vi "Y_AxisMotorControlSetupAndHome.vi"(9 "Serial Settings":T1={"baud rate"=57600, "data bits"=8, "parity"=enum."None", "stop bits"=10, "flow control"=0} {"flow control" items=["None"=0, "XON/XOFF"=1, "RTS/CTS"=2, "DTR/DSR"=4]; "stop bits" items=["1.0"=10, "1.5"=15, "2.0"=20]; "data bits" min=5 max=8 step=1; "baud rate" items=["75"=75, "110"=110, "134"=134, "150"=150, "300"=300, "600"=600, "1200"=1200, "1800"=1800, "2400"=2400, "4800"=4800, "7200"=7200, "9600"=9600, "14400"=14400, "19200"=19200, "28800"=28800, "38400"=38400, "56000"=56000, "57600"=57600, "115200"=115200, "128000"=128000, "230400"=230400]}, 11 "VISA Refnum in":refnum<visa-resource-name>="COM3") -> ()   [LabVIEW 2020]
uses:
  C:/Program Files/National Instruments/LabVIEW 2020/examples/Instrument IO/Serial/support/Serial - Settings.ctl
  <vilib>/Instr/_visa.llb/VISA Configure Serial Port (Instr).vi
panel:
  out "Finished":bool
  out "Status Array":bool[](array[boolean])
  out "Limit Switch Status":i32 format="%b"
  out "Buffer":string
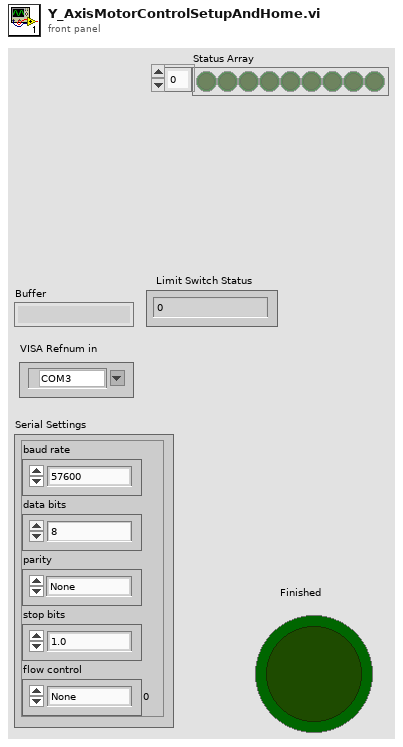
[diagram p1: front panel]
types:
  T1 = typedef "Serial - Settings.ctl" = cluster{"baud rate":u32, "data bits":u16, "parity":enum16{"None", "Odd", "Even", "Mark", "Space"}, "stop bits":u16, "flow control":u16}
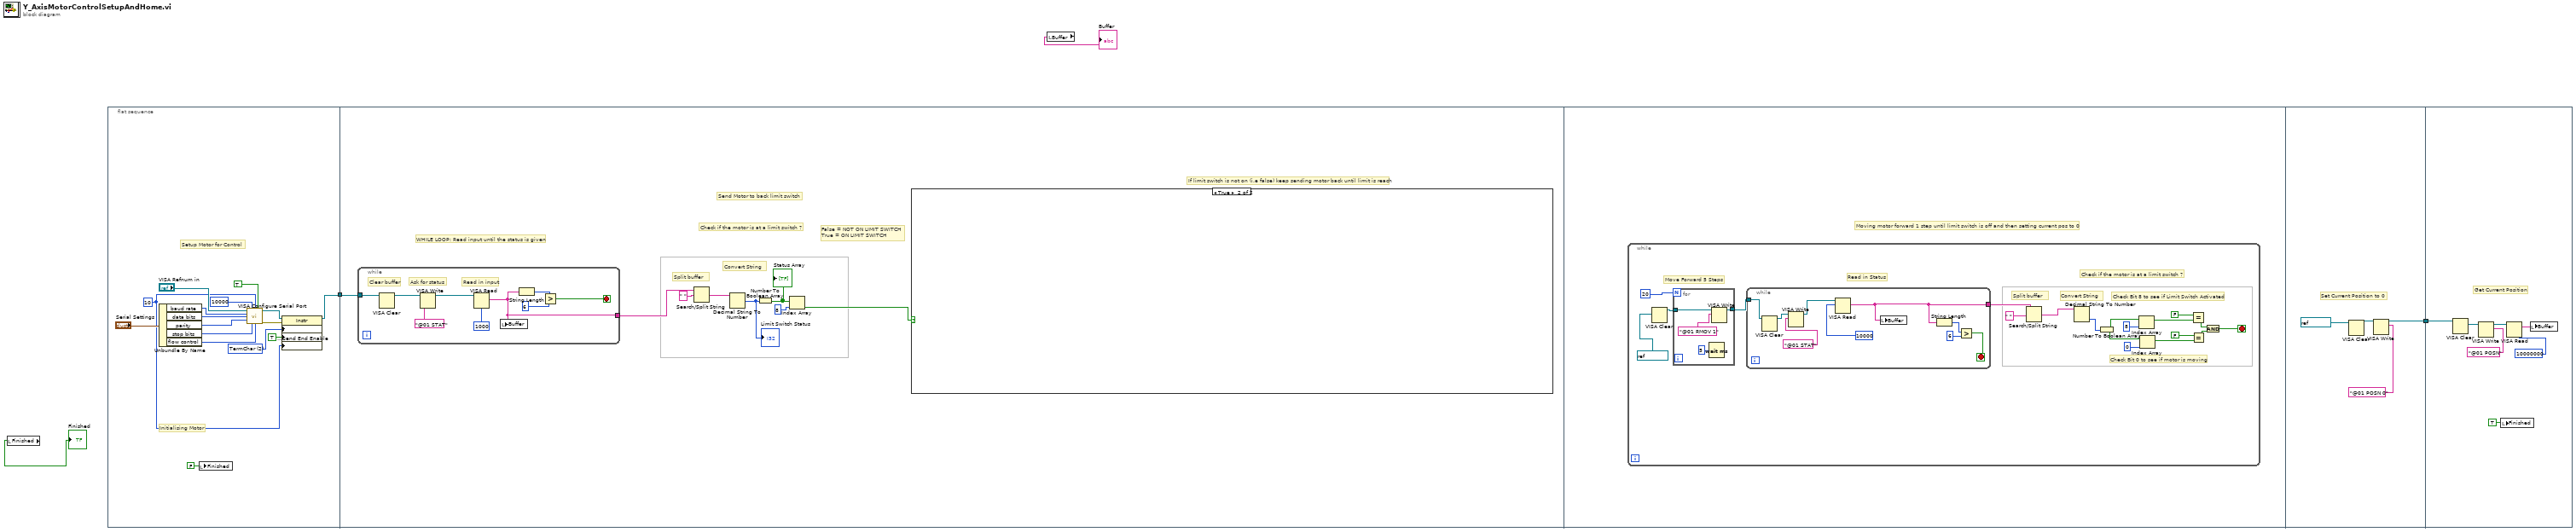
[diagram p0: block diagram]
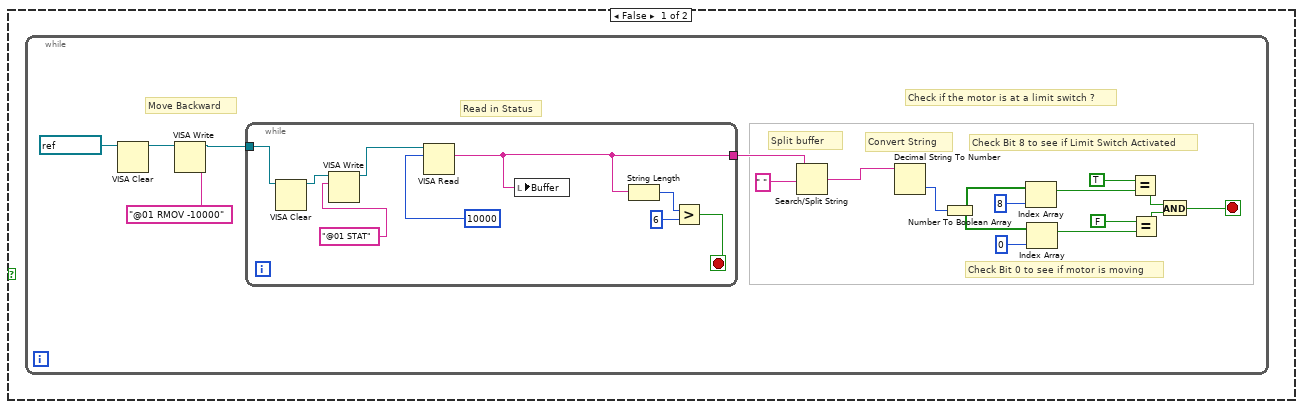
[diagram p2: hidden frame]
diagram:
  n1 = local read "Finished"() -> (→"Finished":bool)
  n2 = flat-sequence {
    tunnel: [w6] -> w4
    tunnel: w4 -> [w22]
    tunnel: [w96] -> w2
    tunnel: w2 -> [w101]
    frame #0 {
      w7 = u8 10 ("Termination Character")
      w11 = u16 2 items=["None", "LastBit", "TermChar", "Break"] ("Serial Settings:Serial End Mode for Writes")
      # "Setup Motor for Control"
      # "Initialising Motor"
      n3 = Unbundle By Name("Serial Settings") -> ("baud rate"=w16:u32, "data bits"=w17:u16, "parity"=w18:enum16{"None", "Odd", "Even", "Mark", "Space"}, "stop bits"=w19:u16, "flow control"=w14:u16)
      n4 = local write "Finished"(FALSE ("Finished")) -> ()
      n5 = call-poly "VISA Configure Serial Port"("VISA resource name"="VISA Refnum in", "timeout (10sec)"=u32 10000, "termination char\n(0xA = '\\n' = LF)"=w7, "Enable Termination\nChar (T)"=TRUE ("End Read on Termination Character?"), "baud rate (9600)"=w16, "data bits (8)"=w17, "parity (0:none)"=w18, "stop bits (10: 1 bit)"=w19, "flow control (0:none)"=w14) -> ("VISA resource name out"=w13:refnum<visa-resource-name>, "error out"=w12:errorcluster)  [unwired: 1 in, 4 out]
      n6 = property class="Instr"(reference=w13, error in=w12, "Serial Settings:End Mode for Writes"=w11, "Message Based Settings:Send End Enable"=TRUE, "Message Based Settings:Termination Character"=w7) -> (reference out=w6:refnum<visa-resource-name>)  [unwired: 1 out]
    }
    frame #1 {
      # "If limit switch is not on (i.e false) keep sending motor back until limit is reach"
      # "Send Motor to back limit switch"
      # "False = NOT ON LIMIT SWITCH \nTrue = ON LIMIT SWITCH"
      # "WHILE LOOP: Read input until the status is given"
      # "Check if the motor is at a limit switch ?"
      # "Convert String"
      # "Split buffer"
      n7 = while {
        tunnel: [w63] -> w24
        tunnel: w22 -> [w58]
        stop <- w59 stop-if-true
        # "Clear buffer"
        # "Ask for status"
        # "Read in input"
        n8 = VISA Clear(VISA resource name=w58) -> (VISA resource name out=w56:refnum<visa-resource-name>)  [unwired: 1 in, 1 out]
        n9 = VISA Write(VISA resource name=w56, write buffer="@01 STAT" ("Command 2")) -> (VISA resource name out=w57:refnum<visa-resource-name>)  [unwired: 1 in, 2 out]
        n10 = VISA Read(VISA resource name=w57, byte count=u32 1000 ("Read Word Length Count?")) -> (read buffer=w63:string)  [unwired: 1 in, 3 out]
        n11 = local write "Buffer"(w63) -> ()
        n12 = String Length(string=w63) -> (length=w62:i32)
        n13 = Greater?(x=w62, y=6) -> (0:w59:bool)
      }
      n14 = Search/Split String(string=w24, search string/char (-)=" ") -> (match + rest of string=w27:string)  [unwired: 1 in, 2 out]
      n15 = Decimal String To Number(string=w27) -> (number=w23:i32)  [unwired: 2 in, 1 out]
      "Limit Switch Status" <- w23
      n16 = Number To Boolean Array(number=w23) -> (Boolean array=w28:bool[])
      "Status Array" <- w28
      n17 = Index Array(array=w28, index=8) -> (element=w21:bool)
      n18 = case shown="True" w21 {
        frame False {
          n19 = while {
            stop <- w37 stop-if-true
            # "Check Bit 0 to see if motor is moving"
            # "Check if the motor is at a limit switch ?"
            # "Read in Status"
            # "Move Backward"
            # "Check Bit 8 to see if Limit Switch Activated"
            # "Convert String"
            # "Split buffer"
            n20 = VISA Clear(VISA resource name=refnum<visa-resource-name> "COM3" ("VISA resource name out")) -> (VISA resource name out=w30:refnum<visa-resource-name>)  [unwired: 1 in, 1 out]
            n21 = VISA Write(VISA resource name=w30, write buffer="@01 RMOV -10000" ("Command 2")) -> (VISA resource name out=w38:refnum<visa-resource-name>)  [unwired: 1 in, 2 out]
            n22 = while {
              tunnel: [w52] -> w41
              tunnel: w38 -> [w47]
              stop <- w51 stop-if-true
              n23 = VISA Clear(VISA resource name=w47) -> (VISA resource name out=w48:refnum<visa-resource-name>)  [unwired: 1 in, 1 out]
              n24 = VISA Write(VISA resource name=w48, write buffer="@01 STAT" ("Command 2")) -> (VISA resource name out=w50:refnum<visa-resource-name>)  [unwired: 1 in, 2 out]
              n25 = VISA Read(VISA resource name=w50, byte count=u32 10000 ("Read Word Length Count?")) -> (read buffer=w52:string)  [unwired: 1 in, 3 out]
              n26 = local write "Buffer"(w52) -> ()
              n27 = String Length(string=w52) -> (length=w54:i32)
              n28 = Greater?(x=w54, y=6) -> (0:w51:bool)
            }
            n29 = Search/Split String(string=w41, search string/char (-)=" ") -> (match + rest of string=w44:string)  [unwired: 1 in, 2 out]
            n30 = Decimal String To Number(string=w44) -> (number=w45:i32)  [unwired: 2 in, 1 out]
            n31 = Number To Boolean Array(number=w45) -> (Boolean array=w32:bool[])
            n32 = Index Array(array=w32, index=8) -> (element=w40:bool)
            n33 = Index Array(array=w32, index=0) -> (element=w34:bool)
            n34 = Equal?(x=TRUE, y=w40) -> (x = y?=w36:bool)
            n35 = Equal?(x=FALSE, y=w34) -> (x = y?=w31:bool)
            n36 = And(x=w36, y=w31) -> (x .and. y?=w37:bool)
          }
        }
        frame True {
        }
      }
    }
    frame #2 {
      # "Moving motor forward 1 step until limit switch is off and then setting current pos to 0"
      n37 = while {
        stop <- w75 stop-if-true
        # "Check Bit 0 to see if motor is moving"
        # "Check if the motor is at a limit switch ?"
        # "Read in Status"
        # "Move Forward 5 Steps"
        # "Check Bit 8 to see if Limit Switch Activated"
        # "Convert String"
        # "Split buffer"
        n38 = VISA Clear(VISA resource name=refnum<visa-resource-name> "COM3" ("VISA resource name out")) -> (VISA resource name out=w66:refnum<visa-resource-name>)  [unwired: 1 in, 1 out]
        n39 = for {
          N: 20 -> [_]
          tunnel: [w85] -> w68
          tunnel: w66 -> [w83]
          n40 = Wait (ms)(milliseconds to wait=u32 5) -> ()  [unwired: 1 out]
          n41 = VISA Write(VISA resource name=w83, write buffer="@01 RMOV 1" ("Command 2")) -> (VISA resource name out=w85:refnum<visa-resource-name>)  [unwired: 1 in, 2 out]
        }
        n42 = while {
          tunnel: [w92] -> w78
          tunnel: w68 -> [w87]
          stop <- w91 stop-if-true
          n43 = VISA Clear(VISA resource name=w87) -> (VISA resource name out=w88:refnum<visa-resource-name>)  [unwired: 1 in, 1 out]
          n44 = VISA Write(VISA resource name=w88, write buffer="@01 STAT" ("Command 2")) -> (VISA resource name out=w90:refnum<visa-resource-name>)  [unwired: 1 in, 2 out]
          n45 = VISA Read(VISA resource name=w90, byte count=u32 10000 ("Read Word Length Count?")) -> (read buffer=w92:string)  [unwired: 1 in, 3 out]
          n46 = local write "Buffer"(w92) -> ()
          n47 = String Length(string=w92) -> (length=w94:i32)
          n48 = Greater?(x=w94, y=6) -> (0:w91:bool)
        }
        n49 = Search/Split String(string=w78, search string/char (-)=" ") -> (match + rest of string=w81:string)  [unwired: 1 in, 2 out]
        n50 = Decimal String To Number(string=w81) -> (number=w82:i32)  [unwired: 2 in, 1 out]
        n51 = Number To Boolean Array(number=w82) -> (Boolean array=w70:bool[])
        n52 = Index Array(array=w70, index=8) -> (element=w77:bool)
        n53 = Index Array(array=w70, index=0) -> (element=w72:bool)
        n54 = Equal?(x=FALSE, y=w77) -> (x = y?=w74:bool)
        n55 = Equal?(x=FALSE, y=w72) -> (x = y?=w69:bool)
        n56 = And(x=w74, y=w69) -> (x .and. y?=w75:bool)
      }
    }
    frame #3 {
      # "Set Current Position to 0"
      n57 = VISA Clear(VISA resource name=refnum<visa-resource-name> "COM3" ("VISA resource name out")) -> (VISA resource name out=w99:refnum<visa-resource-name>)  [unwired: 1 in, 1 out]
      n58 = VISA Write(VISA resource name=w99, write buffer="@01 POSN 0" ("Command 2")) -> (VISA resource name out=w96:refnum<visa-resource-name>)  [unwired: 1 in, 2 out]
    }
    frame #4 {
      # "Get Current Position"
      n59 = VISA Clear(VISA resource name=w101) -> (VISA resource name out=w104:refnum<visa-resource-name>)  [unwired: 1 in, 1 out]
      n60 = VISA Write(VISA resource name=w104, write buffer="@01 POSN" ("Command 2")) -> (VISA resource name out=w105:refnum<visa-resource-name>)  [unwired: 1 in, 2 out]
      n61 = local write "Finished"(TRUE ("Finished")) -> ()
      n62 = VISA Read(VISA resource name=w105, byte count=u32 10000000 ("Read Word Length Count?")) -> (read buffer=w106:string)  [unwired: 1 in, 3 out]
      n63 = local write "Buffer"(w106) -> ()
    }
  }
  n64 = local read "Buffer"() -> (→"Buffer":string)
